vi "TOML example write section.vi"() -> ()   [LabVIEW 2017]
doc: "This example VI demonstrates how to use the TOML library"
uses:
  3dd03dea-ebb6-4d13-ba4c-6119dc4e11fd.vi
  lib/TOML to LabVIEW.vi
  lib/TOML.lvlib
panel:
  out "error":errorcluster caption="LV to TOML error"
  out "TOML to LV error":errorcluster
  in  "support-path":cluster{"file-windows":path, "file-linux":path}
  in  "clients":cluster{"hosts":string[], "data":string[][]}
  in  "database":T1
  in  "Fail":bool
  out "toml":string caption="new TOML String"
  in  "original TOML String":string
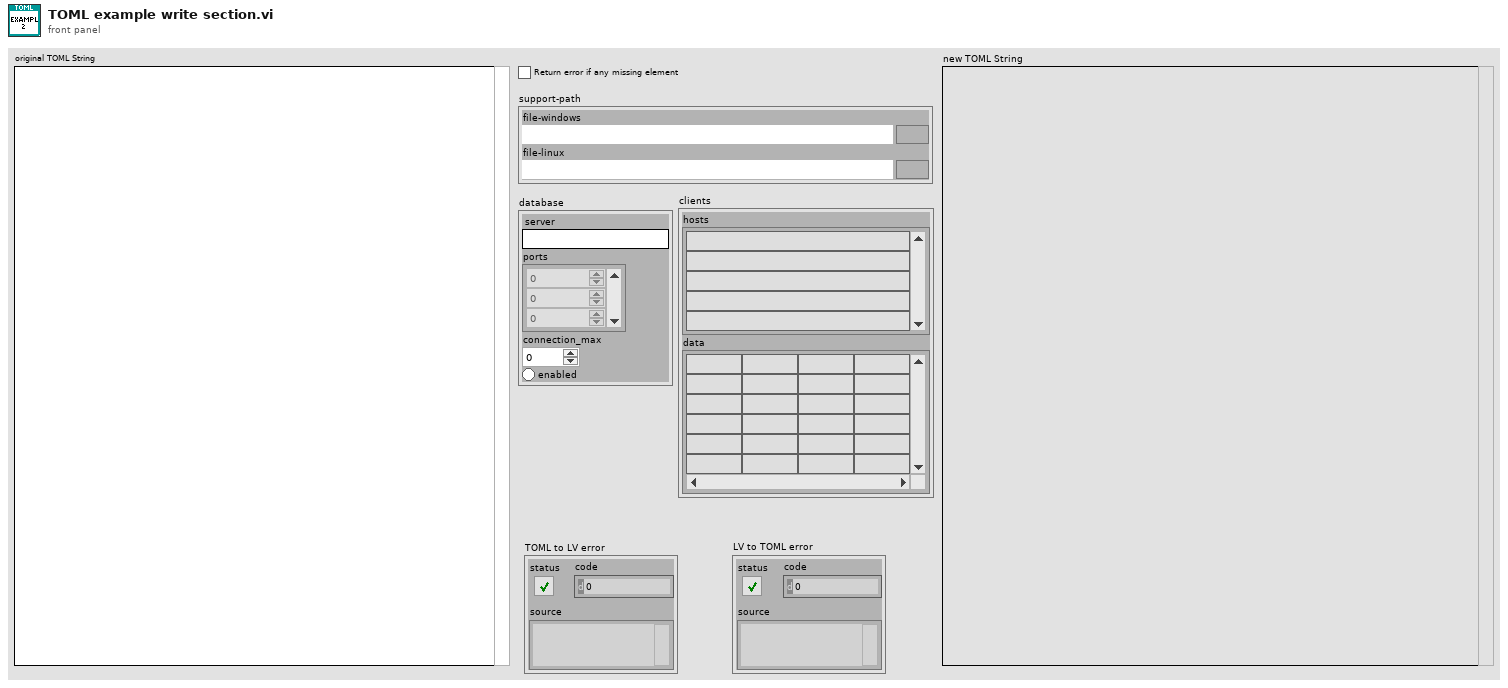
[diagram p1: front panel]
types:
  T1 = cluster{"server":string, "ports":u16[], "connection_max":dbl, "enabled":bool}
  T2 = cluster{"database":cluster{"server":string, "ports":u16[], "connection_max":dbl, "enabled":bool}, "clients":cluster{"hosts":string[], "data":string[][]}, "support-path":cluster{"file-windows":path, "file-linux":path}}
  T3 = typedef "TOML.lvlib/TOML Value.ctl" = cluster{"type":enum16{"Table", "Array", "String", "Integer", "Float", "Boolean", "Offset Date-Time", "Local Date-Time", "Local Date", "Local Time", "Path"}, "value":variant}
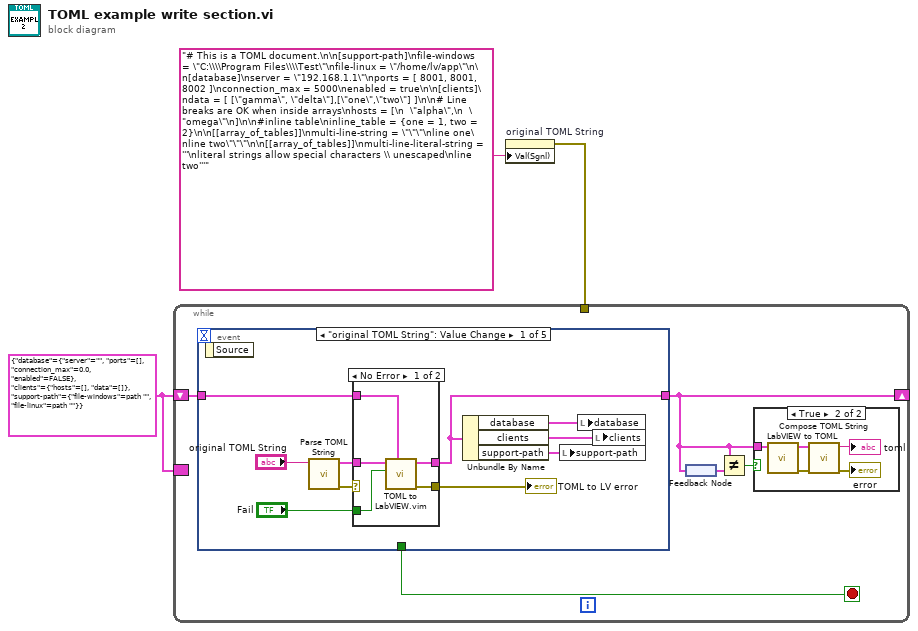
[diagram p0: block diagram]
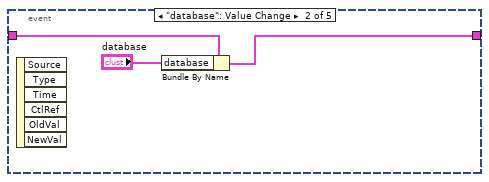
[diagram p4: hidden frame]
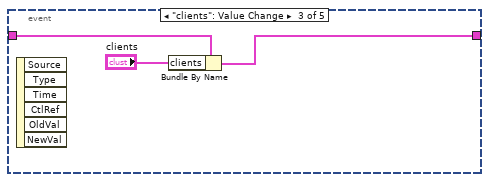
[diagram p5: hidden frame]
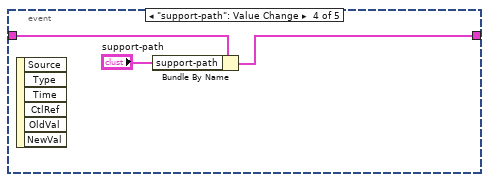
[diagram p6: hidden frame]
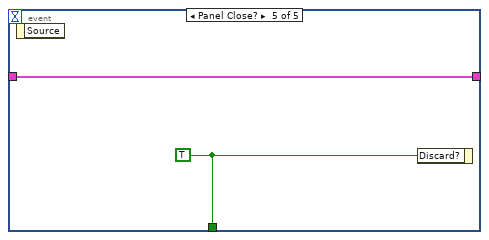
[diagram p7: hidden frame]
diagram:
  w1 = T2 {"database"={"server"="", "ports"=[], "connection_max"=0.0, "enabled"=FALSE}, "clients"={"hosts"=[], "data"=[]}, "support-path"={"file-windows"=path "", "file-linux"=path ""}} ("Parsed Data")
  n1 = property on="original TOML String" class="Str"("Val(Sgnl)"="# This is a TOML document.\n\n[support-path]\nfile-windows = \"C:\\\\Program Files\\\\Test\"\nfile-linux = \"/home/lv/app\"\n\n[database]\nserver = \"192.168.1.1\"\nports = [ 8001, 8001, 8002 ]\nconnection_max = 5000\nenabled = true\n\n[clients]\ndata = [ [\"gamma\", \"delta\"],[\"one\",\"two\"] ]\n\n# Line breaks are OK when inside arrays\nhosts = [\n  \"alpha\",\n  \"omega\"\n]\n\n#inline table\ninline_table = {one = 1, two = 2}\n\n[[array_of_tables]]\nmulti-line-string = \"\"\"\nline one\nline two\"\"\"\n\n[[array_of_tables]]\nmulti-line-literal-string = '''\nliteral strings allow special characters \\ unescaped\nline two'''" ("TOML String")) -> (error out=w2:errorcluster)  [unwired: 2 in, 1 out]
  n2 = while {
    tunnel: w2 -> [_]
    shift-right: [w5] -> _
    shift-left: w1 -> [w7]
    border: w1 -> [_]
    stop <- w8 stop-if-true
    n3 = event shown="[0] \"original TOML String\": Value Change" {
      selector: _ -> [_ _ _ _ _]
      dyn-events: _ -> [_ _ _ _ _]
      timeout: _ -> [_ _ _ _ _]
      tunnel: [_ _ _ _ w40] -> w8
      tunnel: w7 -> [w20 w32 w35 w38 w39]
      tunnel: [w18 w31 w34 w37 w39] -> w5
      event "original TOML String": Value Change {
        n4 = event-data() -> ()  [unwired: 1 in, 1 out]
        n5 = call "Parse TOML String.vi"("String"="original TOML String") -> ("error out"=w23:errorcluster, "Value"=w21:T3)  [unwired: 9 in]
        n6 = case shown="No Error" w23 {
          selector: w23 -> [_ w29]
          tunnel: w21 -> [w28 _]
          tunnel: w20 -> [w27 _]
          tunnel: [w26 _] -> w18
          tunnel: "Fail" -> [w25 _]
          tunnel: [w24 w29] -> w14
          frame No Error {
            n7 = call "TOML to LabVIEW.vim"("datatype"=w27, "Error if missing element"=w25, "Value"=w28) -> ("error out"=w24:errorcluster, "LV Data"=w26:T2)  [unwired: 6 in, 1 out]
          }
          frame Error {
          }
        }
        "TOML to LV error" <- w14
        n8 = Unbundle By Name(w18) -> ("database"=w17:T1, "clients"=w16:cluster{"hosts":string[], "data":string[][]}, "support-path"=w15:cluster{"file-windows":path, "file-linux":path})
        n9 = local write "support-path"(w15) -> ()
        n10 = local write "database"(w17) -> ()
        n11 = local write "clients"(w16) -> ()
      }
      event "database": Value Change {
        n12 = event-data() -> ()  [unwired: 1 in, 6 out]
        n13 = Bundle By Name(cluster=w32, "database"="database") -> (w31:T2)
      }
      event "clients": Value Change {
        n14 = event-data() -> ()  [unwired: 1 in, 6 out]
        n15 = Bundle By Name(cluster=w35, "clients"="clients") -> (w34:T2)
      }
      event "support-path": Value Change {
        n16 = event-data() -> ()  [unwired: 1 in, 6 out]
        n17 = Bundle By Name(cluster=w38, "support-path"="support-path") -> (w37:T2)
      }
      event Panel Close? {
        w40 = TRUE
        n18 = event-data() -> ()  [unwired: 1 in, 1 out]
        n19 = event-data("Discard?"=w40) -> ()  [unwired: 1 in, 1 out]
      }
    }
    n20 = feedback-in #1(w5) -> ()
    n21 = feedback #1() -> (w6:T2)
    n22 = Not Equal?(x=w5, y=w6) -> (x != y?=w4:bool)
    n23 = case shown="True" w4 {
      tunnel: w5 -> [_ w11]
      frame False {
      }
      frame True {
        n24 = call "LabVIEW to TOML.vi"("LV Value"=w11) -> ("error out"=w10:errorcluster, "TOML Value"=w12:T3)  [unwired: 9 in]
        n25 = call "Compose TOML String.vi"("error in (no error)"=w10, "Value"=w12) -> ("error out"=→"error":errorcluster, "String"=→"toml":string)  [unwired: 8 in]
      }
    }
  }
